vi "HMP2020_Manual.vi"(8 "error in (no error)":errorcluster, 11 "HMP4040 VISA":refnum<visa-resource-name>="HMP4040_FTS2") -> (0 "error out":errorcluster, 3 "HMP VISA Out":refnum<visa-resource-name> caption="VISA resource name out")   [LabVIEW 2022 SP3]
uses:
  HMP4040_ChannelControl.ctl
panel:
  out "CH1 Voltage":dbl(knob) caption="Voltage Value" scale=0.0..30.0
  out "CH1 Current":dbl(knob) caption="Current" scale=0.0..3.0
  in  "Control Power":bool
  in  "DC Bus":bool
  out "CH2 Voltage":dbl(knob) caption="Voltage Value" scale=0.0..30.0
  out "CH2 Current":dbl(knob) caption="Current" scale=0.0..3.0
  in  "stop":bool
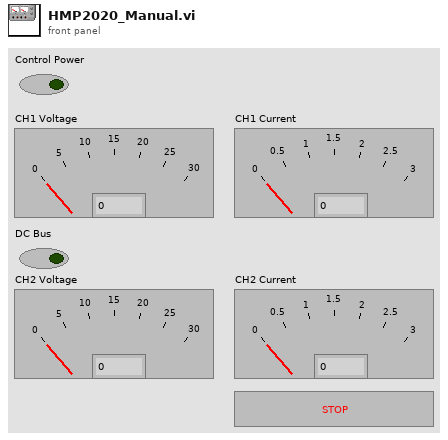
[diagram p1: front panel]
types:
  T1 = typedef "HMP4040_ChannelControl.ctl" = cluster{"CH1 Voltage":dbl, "CH1 Current":dbl, "CH1 Output":bool, "CH2 Voltage":dbl, "CH2 Current":dbl, "CH2 Output":bool, "CH3 Voltage":dbl, "CH3 Current":dbl, "CH3 Output":bool, "CH4 Voltage":dbl, "CH4 Current":dbl, "CH4 Output":bool, "Master Output":bool}
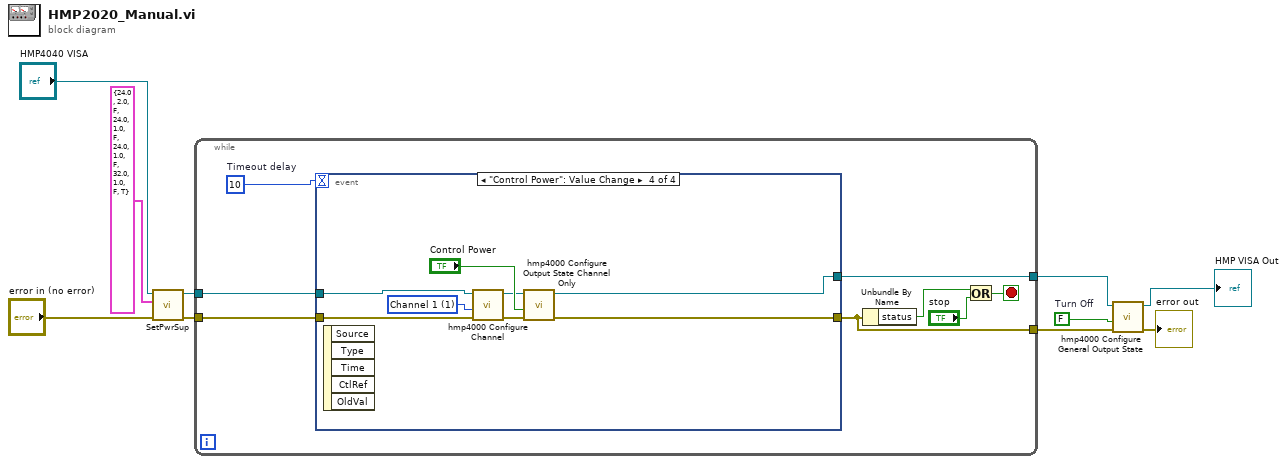
[diagram p0: block diagram]
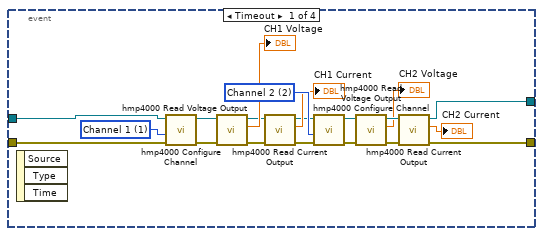
[diagram p2: hidden frame]
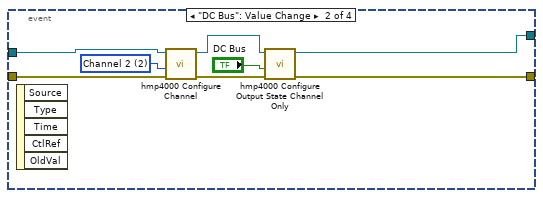
[diagram p3: hidden frame]
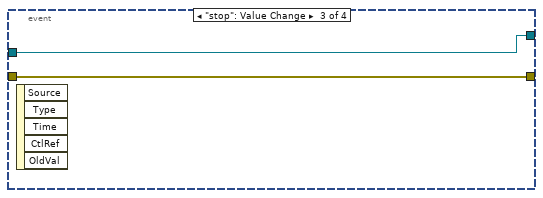
[diagram p4: hidden frame]
diagram:
  w8 = FALSE  # Turn Off
  n1 = call "SetPwrSup.vi"("error in (no error)"="error in (no error)", "HMP4040 Channel Settings"=T1 {"CH1 Voltage"=24.0, "CH1 Current"=2.0, "CH1 Output"=FALSE, "CH2 Voltage"=24.0, "CH2 Current"=1.0, "CH2 Output"=FALSE, "CH3 Voltage"=24.0, "CH3 Current"=1.0, "CH3 Output"=FALSE, "CH4 Voltage"=32.0, "CH4 Current"=1.0, "CH4 Output"=FALSE, "Master Output"=TRUE}, "HMP4040 IN"="HMP4040 VISA") -> ("error out"=w6:errorcluster, "HMP4040_OUT"=w2:refnum<visa-resource-name>)  [unwired: 7 in]
  n2 = while {
    tunnel: w6 -> [w14]
    tunnel: w2 -> [w18]
    tunnel: [w12] -> w7
    tunnel: [w16] -> w9
    stop <- w17 stop-if-true
    w15 = 10  # Timeout delay
    n3 = event shown="[3] \"Control Power\": Value Change" {
      selector: _ -> [_ _ _ _]
      dyn-events: _ -> [_ _ _ _]
      timeout: w15 -> [_ _ _ _]
      tunnel: [w35 w41 w47 w55] -> w12
      tunnel: w14 -> [w21 w42 w48 w49]
      tunnel: w18 -> [w22 w43 w47 w52]
      tunnel: [w36 w40 w48 w56] -> w16
      event Timeout {
        w27 = 1 items=["Channel 1"=1, "Channel 2"=2, "Channel 3"=3, "Channel 4"=4] ("Channel (Channel 1)")
        w32 = 2 items=["Channel 1"=1, "Channel 2"=2, "Channel 3"=3, "Channel 4"=4] ("Channel (Channel 1)")
        n4 = event-data() -> ()  [unwired: 1 in, 3 out]
        n5 = call "hmp4000 Configure Channel.vi"("error in (no error)"=w21, "Channel (Channel 1)"=w27, "VISA resource name"=w22) -> ("error out"=w29:errorcluster, "VISA resource name out"=w28:refnum<visa-resource-name>)  [unwired: 7 in]
        n6 = call "hmp4000 Read Voltage Output.vi"("error in (no error)"=w29, "VISA resource name"=w28) -> ("error out"=w24:errorcluster, "Voltage Value"=→"CH1 Voltage":dbl, "VISA resource name out"=w23:refnum<visa-resource-name>)  [unwired: 7 in]
        n7 = call "hmp4000 Read Current Output.vi"("error in (no error)"=w24, "VISA resource name"=w23) -> ("error out"=w19:errorcluster, "Current Value"=→"CH1 Current":dbl, "VISA resource name out"=w20:refnum<visa-resource-name>)  [unwired: 7 in]
        n8 = call "hmp4000 Configure Channel.vi"("error in (no error)"=w19, "Channel (Channel 1)"=w32, "VISA resource name"=w20) -> ("error out"=w30:errorcluster, "VISA resource name out"=w31:refnum<visa-resource-name>)  [unwired: 7 in]
        n9 = call "hmp4000 Read Voltage Output.vi"("error in (no error)"=w30, "VISA resource name"=w31) -> ("error out"=w37:errorcluster, "Voltage Value"=→"CH2 Voltage":dbl, "VISA resource name out"=w38:refnum<visa-resource-name>)  [unwired: 7 in]
        n10 = call "hmp4000 Read Current Output.vi"("error in (no error)"=w37, "VISA resource name"=w38) -> ("error out"=w36:errorcluster, "Current Value"=→"CH2 Current":dbl, "VISA resource name out"=w35:refnum<visa-resource-name>)  [unwired: 7 in]
      }
      event "DC Bus": Value Change {
        w46 = 2 items=["Channel 1"=1, "Channel 2"=2, "Channel 3"=3, "Channel 4"=4] ("Channel (Channel 1)")
        n11 = event-data() -> ()  [unwired: 1 in, 5 out]
        n12 = call "hmp4000 Configure Channel.vi"("error in (no error)"=w42, "Channel (Channel 1)"=w46, "VISA resource name"=w43) -> ("error out"=w44:errorcluster, "VISA resource name out"=w45:refnum<visa-resource-name>)  [unwired: 7 in]
        n13 = call "hmp4000 Configure Output State Channel Only.vi"("error in (no error)"=w44, "Output State (Off)"="DC Bus", "VISA resource name"=w45) -> ("error out"=w40:errorcluster, "VISA resource name out"=w41:refnum<visa-resource-name>)  [unwired: 7 in]
      }
      event "stop": Value Change {
        n14 = event-data() -> ()  [unwired: 1 in, 5 out]
      }
      event "Control Power": Value Change {
        w53 = 1 items=["Channel 1"=1, "Channel 2"=2, "Channel 3"=3, "Channel 4"=4] ("Channel (Channel 1)")
        n15 = event-data() -> ()  [unwired: 1 in, 5 out]
        n16 = call "hmp4000 Configure Channel.vi"("error in (no error)"=w49, "Channel (Channel 1)"=w53, "VISA resource name"=w52) -> ("error out"=w50:errorcluster, "VISA resource name out"=w51:refnum<visa-resource-name>)  [unwired: 7 in]
        n17 = call "hmp4000 Configure Output State Channel Only.vi"("error in (no error)"=w50, "Output State (Off)"="Control Power", "VISA resource name"=w51) -> ("error out"=w56:errorcluster, "VISA resource name out"=w55:refnum<visa-resource-name>)  [unwired: 7 in]
      }
    }
    n18 = Unbundle By Name(w16) -> ("status"=w13:bool)
    n19 = Or(x=w13, y="stop") -> (x .or. y?=w17:bool)
  }
  n20 = call "hmp4000 Configure General Output State.vi"("error in (no error)"=w9, "Output State (Off)"=w8, "VISA resource name"=w7) -> ("error out"=→"error out":errorcluster, "VISA resource name out"=→"HMP VISA Out":refnum<visa-resource-name>)  [unwired: 7 in]
